vi "Read.vi"(8 "error in (no error)":errorcluster, 11 "VISA resource name":refnum<visa-resource-name>) -> (0 "error out":errorcluster, 1 "End":bool, 2 "Recibo de Datos":string, 3 "VISA resource name out":refnum<visa-resource-name>)   [LabVIEW 2020, in "Control de MaP.lvlib"]
uses:
  Control de MaP.lvlib
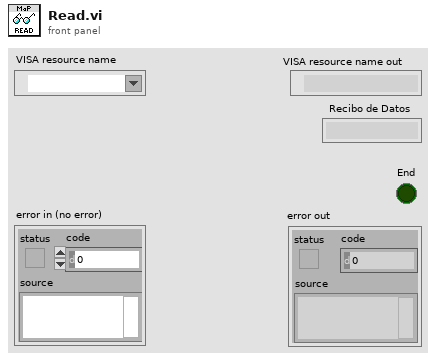
[diagram p1: front panel]
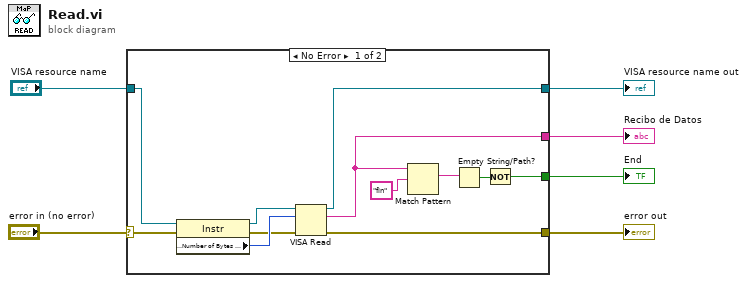
[diagram p0: block diagram]
diagram:
  n1 = case shown="No Error" "error in (no error)" {
    selector: "error in (no error)" -> [w14 w20]
    tunnel: "VISA resource name" -> [w15 w19]
    tunnel: [w13 w19] -> w4
    tunnel: [w12 w20] -> w3
    tunnel: [w11 _] -> w2
    tunnel: [w7 _] -> w1
    frame No Error {
      n2 = property class="Instr"(reference=w15, error in=w14) -> (reference out=w16:refnum<visa-resource-name>, error out=w17:errorcluster, "Serial Settings:Number of Bytes at Serial Port"=w18:u32)
      n3 = VISA Read(VISA resource name=w16, byte count=w18, error in (no error)=w17) -> (VISA resource name out=w13:refnum<visa-resource-name>, read buffer=w11:string, error out=w12:errorcluster)  [unwired: 1 out]
      n4 = Match Pattern(string=w11, regular expression="fin") -> (match substring=w9:string)  [unwired: 1 in, 3 out]
      n5 = Empty String/Path?(string/path=w9) -> (empty?=w8:bool)
      n6 = Not(x=w8) -> (.not. x?=w7:bool)
    }
    frame Error {
    }
  }
  "VISA resource name out" <- w4
  "error out" <- w3
  "Recibo de Datos" <- w2
  "End" <- w1
